vi "SubPanelVI2.vi"() -> ()   [LabVIEW 2016, in "test_ValueSignal.lvlib"]
uses:
  test_ValueSignal.lvlib
panel:
  in  "Stop":bool
  out "Output":string
  in  "Concatenate":bool
  in  "Input":cluster{"Numeric":dbl, "String":string}
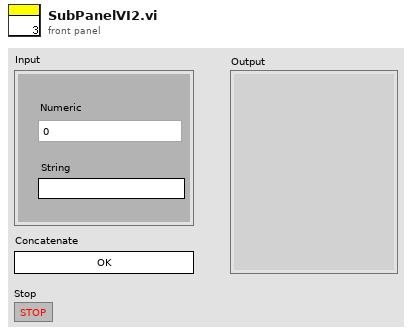
[diagram p1: front panel]
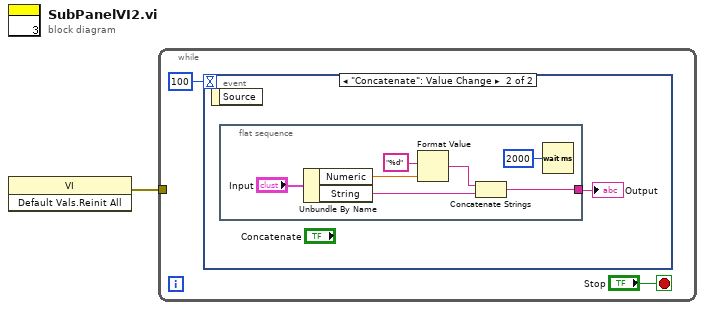
[diagram p0: block diagram]
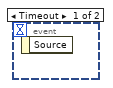
[diagram p2: hidden frame]
diagram:
  n1 = invoke class="VI" method="Default Vals.Reinit All"() -> (error out=w1:errorcluster)  [unwired: 3 in, 2 out]
  n2 = while {
    tunnel: w1 -> [_]
    stop <- "Stop" stop-if-true
    n3 = event shown="[1] \"Concatenate\": Value Change" {
      selector: _ -> [_ _]
      dyn-events: _ -> [_ _]
      timeout: 100 -> [_ _]
      event Timeout {
        n4 = event-data() -> ()  [unwired: 1 in, 1 out]
      }
      event "Concatenate": Value Change {
        n5 = event-data() -> ()  [unwired: 1 in, 1 out]
        n6 = flat-sequence {
          tunnel: [w6] -> w4
          frame #0 {
            n7 = Unbundle By Name("Input") -> ("Numeric"=w10:dbl, "String"=w7:string)
            n8 = Format Value(format string="%d", value (0)=w10) -> (output string=w8:string)  [unwired: 1 in]
            n9 = Concatenate Strings(w8, w7) -> (w6:string)
            n10 = Wait (ms)(milliseconds to wait=u32 2000) -> ()  [unwired: 1 out]
          }
        }
        "Output" <- w4
      }
    }
  }
